vi "Filter Items.vi"(9 "Filter":T1, 11 "Saved VI Data":T4[](array[typedef])) -> (1 "Displayed Indices":i32[](array[numeric]), 3 "Saved VI Data out":T4[](array[typedef]))   [LabVIEW 2023, in "VI Properties Editor.lvlib"]
uses:
  VI Properties Editor.lvlib
  CTLs/VI Data.ctl
  CTLs/VI Properties.ctl
  <vilib>/picture/picture.llb/imagedata.ctl
  CTLs/Control Properties.ctl
  CTLs/Filter.ctl
  CTLs/Filter Column.ctl
  CTLs/Filter Type.ctl
  <vilib>/regexp/Match Regular Expression.xnode
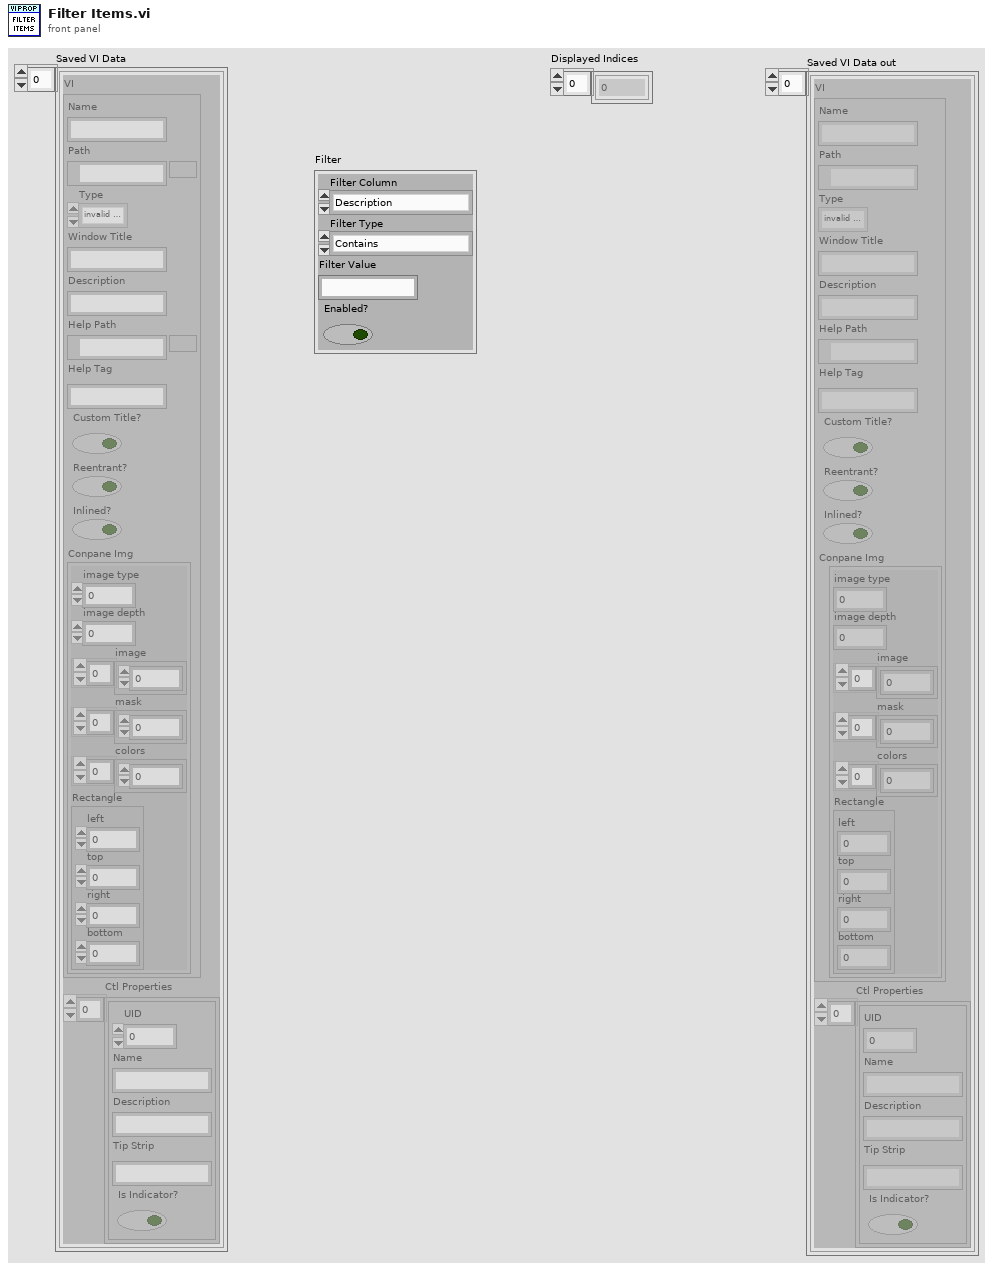
[diagram p1: front panel]
types:
  T1 = typedef "VI Properties Editor.lvlib/Filter.ctl" = cluster{"Filter Column":T2, "Filter Type":T3, "Filter Value":string, "Enabled?":bool}
  T2 = typedef "VI Properties Editor.lvlib/Filter Column.ctl" = enum16{"Description"}
  T3 = typedef "VI Properties Editor.lvlib/Filter Type.ctl" = enum16{"Contains", "Equals", "Starts with", "Ends with", "Does not contain", "Does not equal", "Is empty", "Is not empty"}
  T4 = typedef "VI Properties Editor.lvlib/VI Data.ctl" = cluster{"VI":T5, "Ctl Properties":T7[]}
  T5 = typedef "VI Properties Editor.lvlib/VI Properties.ctl" = cluster{"Name":string, "Path":path, "Type":enum32{"invalid VI type", "Standard VI", "Control VI", "Global VI", "Polymorphic VI", "Configuration VI", "SubSystem", "Facade VI", "Method VI", "Statechart Diagram VI"}, "Window Title":string, "Description":string, "Help Path":path, "Help Tag":string, "Custom Title?":bool, "Reentrant?":bool, "Inlined?":bool, "Conpane Img":T6}
  T6 = typedef "imagedata.ctl" = cluster{"image type":i32, "image depth":i32, "image":u8[], "mask":u8[], "colors":u32[], "Rectangle":cluster{"left":i16, "top":i16, "right":i16, "bottom":i16}}
  T7 = typedef "VI Properties Editor.lvlib/Control Properties.ctl" = cluster{"UID":i32, "Name":string, "Description":string, "Tip Strip":string, "Is Indicator?":bool}
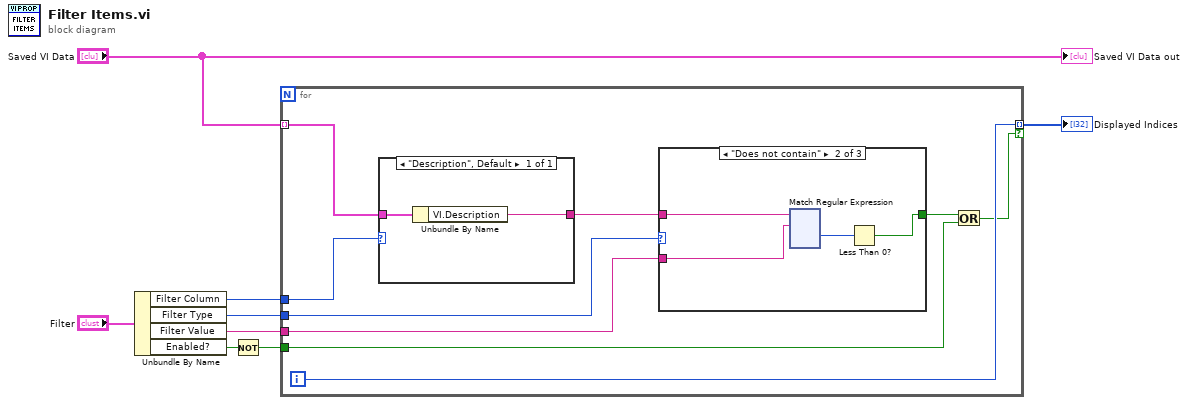
[diagram p0: block diagram]
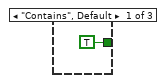
[diagram p2: hidden frame]
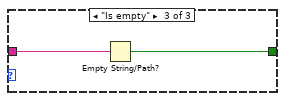
[diagram p3: hidden frame]
diagram:
  n1 = Unbundle By Name("Filter") -> ("Filter Column"=w7:T2, "Filter Type"=w6:T3, "Filter Value"=w5:string, "Enabled?"=w2:bool)
  n2 = Not(x=w2) -> (.not. x?=w1:bool)
  n3 = for {
    tunnel: "Saved VI Data" -> [w13] mode=indexing
    tunnel: w7 -> [w17]
    tunnel: w6 -> [w16]
    tunnel: w5 -> [w15]
    tunnel: [w12] -> w3 mode=indexing if=w10
    tunnel: w1 -> [w9]
    i -> [w12]
    n4 = case shown="\"Description\", Default" w17 {
      tunnel: w13 -> [w143]
      tunnel: [w142] -> w14
      frame "Description", Default {
        n5 = Unbundle By Name(w143) -> ("VI.Description"=w142:string)
      }
    }
    n6 = case shown="\"Does not contain\"" w16 {
      tunnel: w15 -> [_ w21 _]
      tunnel: w14 -> [_ w22 w141]
      tunnel: [TRUE w19 w140] -> w11
      frame "Contains", Default {
      }
      frame "Does not contain" {
        n7 = xnode "Match Regular Expression"("input string"=w22, "regular expression"=w21) -> ("offset past match"=w20:i32)  [unwired: 4 in, 4 out]
        n8 = Less Than 0?(x=w20) -> (x < 0?=w19:bool)
      }
      frame "Is empty" {
        n9 = Empty String/Path?(string/path=w141) -> (empty?=w140:bool)
      }
    }
    n10 = Or(x=w11, y=w9) -> (x .or. y?=w10:bool)
  }
  "Displayed Indices" <- w3
  "Saved VI Data out" <- "Saved VI Data"
